vi "TestPython.vi"   [LabVIEW 2013]
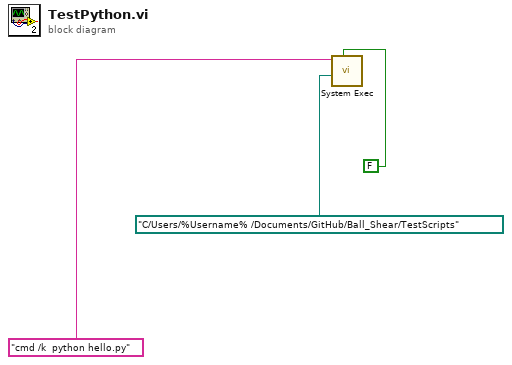
[diagram p0: block diagram]
diagram:
  n1 = call <vilib>:"System Exec.vi"("wait until completion? (T)"=FALSE, "working directory"=path "C:/Users/%Username% /Documents/GitHub/Ball_Shear/TestScripts", "command line"="cmd /k  python hello.py") -> ()  [unwired: 5 in, 4 out]
